vi "_Custom Device Channel.vi"(8 "error in (no error)":errorcluster, 11 "Node Ptr":u64) -> (0 "error out":errorcluster)   [LabVIEW 2020]
uses:
  5565/Source Code/NI VeriStand/Shared/NIVS_Shared.lvlib
  5565/Source Code/NI VeriStand/System Explorer/Communication Layer/Communication.lvlib
  5565/Source Code/NI VeriStand/System Explorer/Communication Layer/FGVActions.ctl
  5565/Source Code/NI VeriStand/Shared/System Storage/Tree Storage/Tree Storage.lvlib
  5565/Source Code/NI VeriStand/System Explorer/System Explorer Framework/System Explorer Framework.lvlib
  5565/Source Code/NI VeriStand/System Explorer/System UI VIs/Custom Device/Custom Device.lvlib
  5565/Source Code/NI VeriStand/Shared/System Storage/Target Sections/Custom Devices/Custom Devices Storage.lvlib
  5565/Source Code/NI VeriStand/Shared/System Storage/Target System Storage/Target System Storage.lvlib
  5565/Source Code/NI VeriStand/Shared/System Storage/Target System Storage/Channel Bitfield Settings.ctl
  5565/Source Code/NI VeriStand/System Explorer/System Explorer Framework/Section Divider.ctl
panel:
  in  "Default Value":dbl
  out "Channel Settings":i32(listbox)
  in  "Channel Settings":T1={"Section Name"="Custom Device Channel Specification"}
  out "Name":string
  in  "Description":string
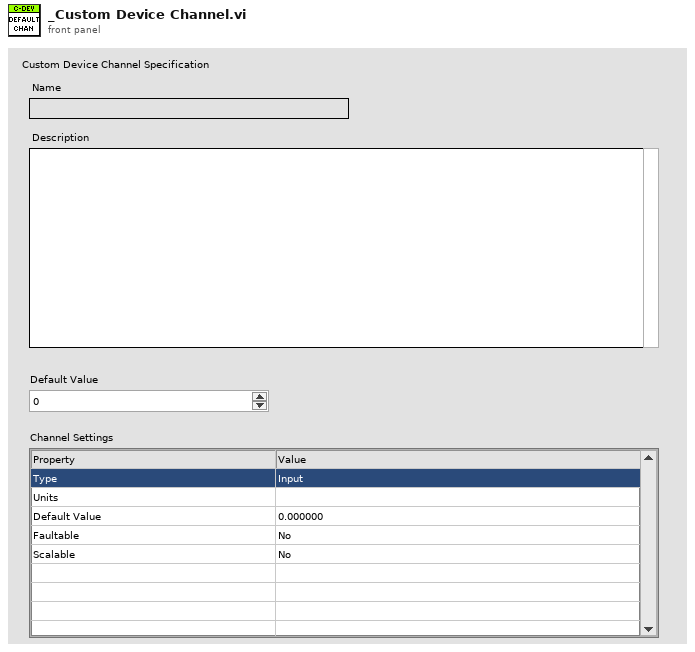
[diagram p1: front panel]
types:
  T1 = typedef "System Explorer Framework.lvlib/Section Divider.ctl" = cluster{"Section Name":string}
  T2 = typedef "Communication.lvlib/FGVActions.ctl" = enum16{"Generate Event", "Get Event Ref", "Create Event", "Destroy"}
  T3 = typedef "NIVS_DataStorage.lvlib/BaseNodeType.ctl" = refnum<k24>
  T4 = typedef "Target System Storage.lvlib/Channel Bitfield Settings.ctl" = enum16{"Read Access", "Write Access", "Faultable", "Scalable"}
  T5 = typedef "Target System Storage.lvlib/Channel Info.ctl" = cluster{"PreScaled Units":string, "Dims":T6, "Def.Value":dbl[], "Bitfield":u32}
  T6 = typedef "Target System Storage.lvlib/Channel Dimensions.ctl" = cluster{"Rows":i32, "Cols":i32}
  T7 = typedef "Communication.lvlib/General Communication Action.ctl" = enum16{"Event structure", "Unsaved", "Release FP Cursor", "Set FP Cursor Busy", "Refresh (Flood)", "Refresh (Add)", "Refresh (Add no highlight)", "Refresh (Repopulate certain node)", "Refresh (Update)", "Refresh (Delete)", "Refresh (Delete no highlight)", "Refresh (Rename)", "Refresh (Move)", "Refresh (Move no highlight)", "Refresh (no highlight)", "Refresh (CD)", "Refresh (single nodes)", "Stop", "GW_WD: Save", "GW_WD: Add Items", "GW_WD: Add Items (no highlight)", "GW_WD: Add Item (CD)", "GW_WD: Update Items", "GW_WD: Delete Item", "GW_WD: Delete Item (no highlight)", "GW_WD: Force Delete Item (no highlight)", "GW_WD: Force Delete Item (no highlight - requested item only)", "GW_WD: Force Delete Item (no highlight - requested item only / Skip Action VI)", "GW_WD: Rename Item", "GW_WD: Move Item", "GW_WD: Repopulate Node", "GW_WD: Load Data from Disk", "GW_WD: Import Data", "GW_WD: New", "GW_WD: Action on Save", "GW_WD: Action on System Shutdown", "GW_WD: Ask save SDF", "GW_WD: Add Revision", "GW_WD: Filter Stop", "GW_WD: Open", "GW_WD: Action on Load", "GW_WD: Save as...", "GW_WD: Deploy", "GW_WD: Close System Explorer", "GW_WD: Current page commit changes", "GW_WD: Current page shutdown", "GW_WD: Add Rev History", "GW_WD: Wait on Action Load", "GW_WD: Signalize Load is Done", "GW_WD: Open File", "GW_WD: Wait on Action Save", "GW_WD: Wait on Action Delete", "GW_WD: Signalize Action Save is Done", "GW_WD: Signalize Action Delete is Done", "GW_WD: Hide Progress Dialog", "GW_WD: Show Progress Dialog", "Delete Cancelled", "GW_WD: Relaunch Page", "GW_WD: Add Item (CD no highlight)", "GW_WD: Activate Progress Window", "GW_WD: Close Progress Window", "GW_WD: Buffering Enabled", "GW_WD: Commit Changes", "GW_WD: Delete Item (notification)", "GW_WD: Force Delete Item (no highlight - notification)", "Page: Send Button ID", "GW_WD: Copy", "GW_WD: Cut", "GW_WD: Paste", "GW_WD: Warning", "GW_WD: Wait on Action Paste", "GW_WD: Signalize Action Paste is Done", "GW_WD: Items Added (highlight)", "GW_WD: Items Added (no highlight)", "GW_WD: Items Added (no highlight / skip action VI)", "GW_WD: Items Added (repopulate certain node)", "GW_WD: Launch Busy Dialog Data Storage", "GW_WD: Stop Busy Dialog Data Storage", "Enable Dynamic Button", "Disable Dynamic Button", "GW_WD: Items Deleted", "GW_WD: Items Deleted (no highlight)", "Insert VI Into SubPanel", "Highlight item", "Update Error Count"}
  T8 = typedef "Communication.lvlib/Listener.ctl" = enum16{"ALL", "System Explorer", "SubPanel VI", "Dialog VI", "Action VI", "GW_WD", "Individual Listener"}
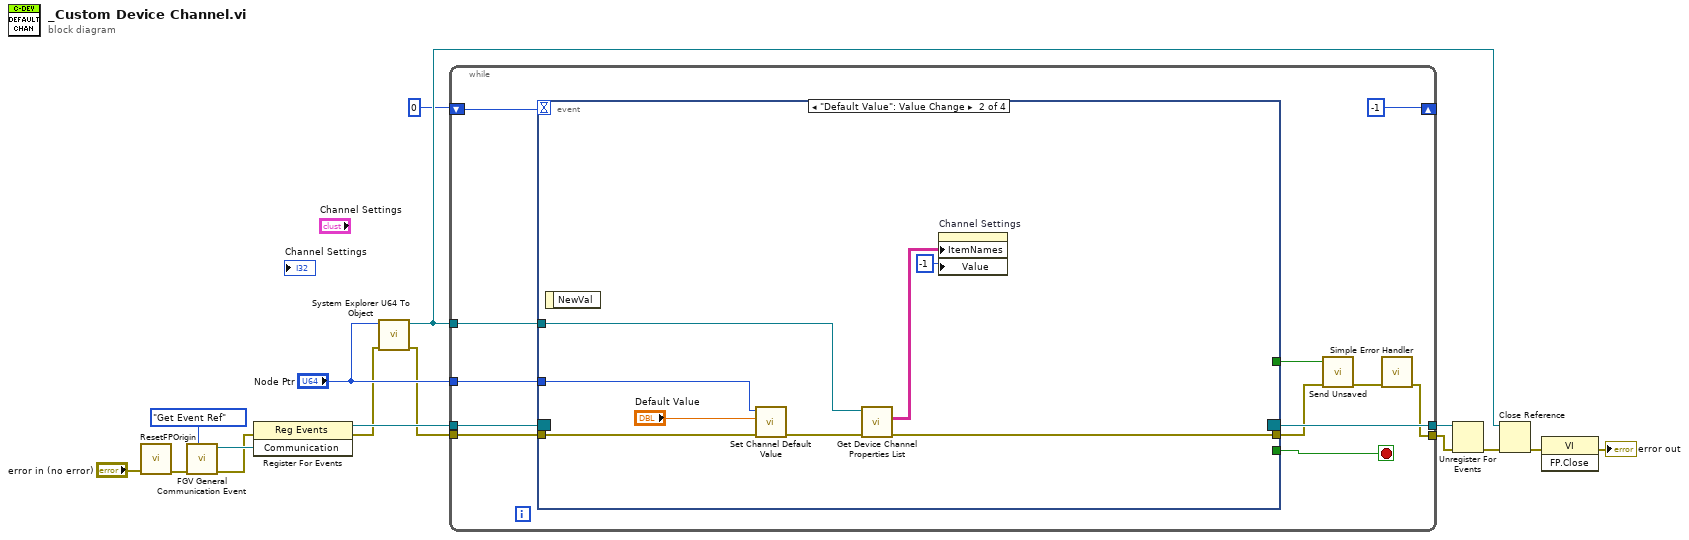
[diagram p0: block diagram]
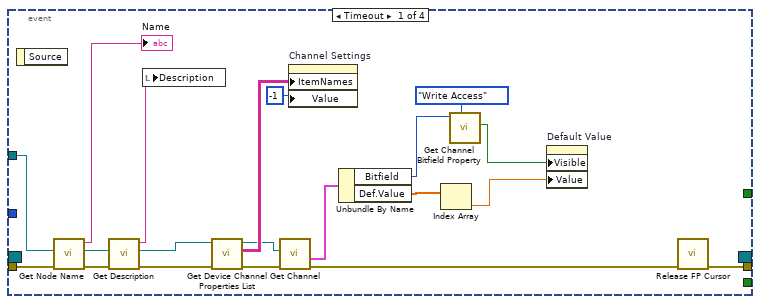
[diagram p2: hidden frame]
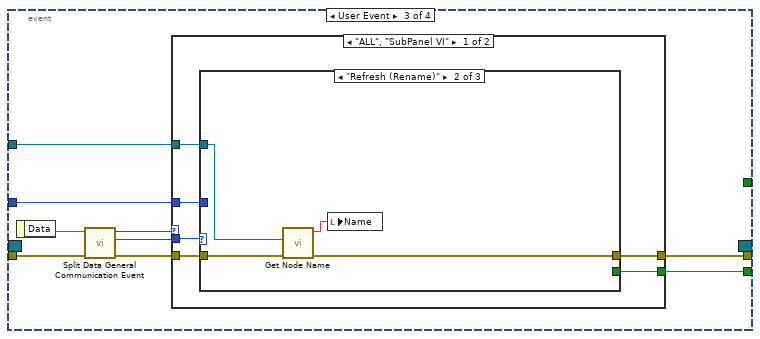
[diagram p3: hidden frame]
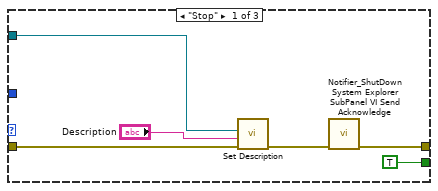
[diagram p4: hidden frame]
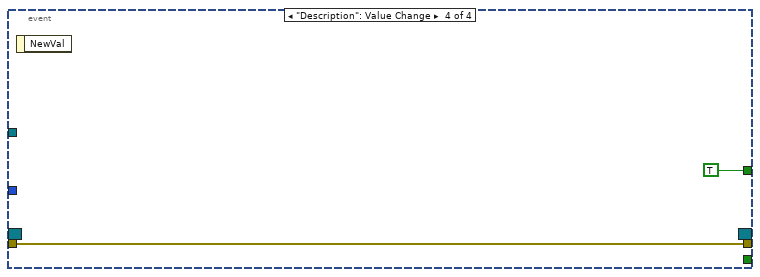
[diagram p7: hidden frame]
diagram:
  n1 = call "ResetFPOrigin.vi"("error in (no error)"="error in (no error)") -> ("error out"=w8:errorcluster)  [unwired: 1 in, 9 out]
  n2 = call "FGV General Communication Event.vi"("Action"=FGVActions."Get Event Ref", "error in (no error)"=w8) -> ("error out"=w11:errorcluster, "Communication"=w12:refnum<user-event>)  [unwired: 1 in, 7 out]
  n3 = register-events(error in=w11, w12) -> (reference out=w10:refnum<event-registration>, error out=w3:errorcluster)  [unwired: 1 in]
  n4 = call "System Explorer U64 To Object.vi"("error in (no error)"=w3, "Node Ptr"="Node Ptr") -> ("error out"=w2:errorcluster, "NodeObject"=w4:T3)  [unwired: 7 in, 1 out]
  n5 = while {
    tunnel: [w28] -> w16
    tunnel: [w27] -> w15
    tunnel: w2 -> [w26]
    tunnel: w10 -> [w25]
    tunnel: "Node Ptr" -> [w23]
    tunnel: w4 -> [w19]
    shift-right: [-1] -> _
    shift-left: 0 -> [w18]
    stop <- w24 stop-if-true
    n6 = event shown="[1] \"Default Value\": Value Change" {
      selector: w25 -> [_ _ _ _]
      dyn-events: [_ _ _ _] -> w28
      timeout: w18 -> [_ _ _ _]
      tunnel: w26 -> [w48 w56 w63 w84]
      tunnel: [_ _ w65 _] -> w24
      tunnel: [w47 w50 w64 w84] -> w21
      tunnel: w23 -> [_ w55 w58 _]
      tunnel: [_ _ _ TRUE] -> w20
      tunnel: w19 -> [w42 w49 w57 _]
      event Timeout {
        n7 = event-data() -> ()  [unwired: 2 out]
        n8 = call "Get Node Name.vi"("error in (no error)"=w48, "BaseNdType"=w42) -> ("error out"=w40:errorcluster, "BaseNdType"=w41:T3, "Node Name"=→"Name":string)  [unwired: 7 out]
        n9 = call "Get Description.vi"("error in (no error)"=w40, "BaseNdType in"=w41) -> ("error out"=w38:errorcluster, "BaseNdType out"=w37:T3, "Description"=w39:string)  [unwired: 6 in, 1 out]
        n10 = local write "Description"(w39) -> ()
        n11 = call "Get Device Channel Properties List.vi"("error in (no error)"=w38, "Channel Ref in"=w37) -> ("error out"=w35:errorcluster, "Properties List"=w44:string[][], "Channel Ref out"=w36:T3)  [unwired: 7 out]
        n12 = call "Get Channel.vi"("error in (no error)"=w35, "Channel"=w36) -> ("error out"=w34:errorcluster, "Channel Info"=w33:T5)  [unwired: 6 in, 2 out]
        n13 = property on="Channel Settings" class="MCListbox (strict)"("ItemNames"=w44, "Value"=-1 ("Channel Settings")) -> ()  [unwired: 2 in, 2 out]
        n14 = Unbundle By Name(w33) -> ("Bitfield"=w30:u32, "Def.Value"=w43:dbl[])
        n15 = Index Array(array=w43) -> (element=w32:dbl)  [unwired: 1 in]
        n16 = call "Get Channel Bitfield Property.vi"("Bitfield Setting"=Channel_Bitfield_Settings."Write Access", "Channel Bitfield"=w30) -> ("Value"=w29:bool)  [unwired: 9 out]
        n17 = property on="Default Value" class="DigNum (strict)"("Visible"=w29, "Value"=w32) -> ()  [unwired: 2 in, 2 out]
        n18 = call "Release FP Cursor.vi"("error in (no error)"=w34) -> ("error out"=w47:errorcluster)  [unwired: 10 out]
      }
      event "Default Value": Value Change {
        n19 = event-data() -> ()  [unwired: 2 out]
        n20 = call "Set Channel Default Value.vi"("error in (no error)"=w56, "Default Value"="Default Value", "Channel Ref in"=w55) -> ("error out"=w51:errorcluster)  [unwired: 8 out]
        n21 = call "Get Device Channel Properties List.vi"("error in (no error)"=w51, "Channel Ref in"=w49) -> ("error out"=w50:errorcluster, "Properties List"=w52:string[][])  [unwired: 8 out]
        n22 = property on="Channel Settings" class="MCListbox (strict)"("ItemNames"=w52, "Value"=-1 ("Channel Settings")) -> ()  [unwired: 2 in, 2 out]
      }
      event User Event {
        n23 = event-data() -> ("Data"=w62:string)  [unwired: 1 out]
        n24 = call "Split Data General Communication Event.vi"("error in"=w63, "Data"=w62) -> ("error out"=w61:errorcluster, "Action"=w59:T7, "Listener"=w60:T8)  [unwired: 7 out]
        n25 = case shown="\"ALL\", \"SubPanel VI\"" w60 {
          tunnel: w61 -> [w70 w83]
          tunnel: w59 -> [w71 _]
          tunnel: [w69 _] -> w65
          tunnel: [w68 w83] -> w64
          tunnel: w58 -> [w67 _]
          tunnel: w57 -> [w66 _]
          frame "ALL", "SubPanel VI" {
            n26 = case shown="\"Refresh (Rename)\"" w71 {
              tunnel: w70 -> [w73 w81 w82]
              tunnel: [w77 w79 w82] -> w68
              tunnel: [TRUE _ _] -> w69
              tunnel: w67 -> [_ _ _]
              tunnel: w66 -> [w75 w78 _]
              frame "Stop" {
                n27 = call "Set Description.vi"("error in (no error)"=w73, "Description"="Description", "BaseNdType in"=w75) -> ("error out"=w72:errorcluster)  [unwired: 6 in, 2 out]
                n28 = call "Notifier_ShutDown System Explorer SubPanel VI Send Acknowledge.vi"("error in (no error)"=w72) -> ("error out"=w77:errorcluster)  [unwired: 1 in, 9 out]
              }
              frame "Refresh (Rename)" {
                n29 = call "Get Node Name.vi"("error in (no error)"=w81, "BaseNdType"=w78) -> ("error out"=w79:errorcluster, "Node Name"=w80:string)  [unwired: 8 out]
                n30 = local write "Name"(w80) -> ()
              }
              frame Default {
              }
            }
          }
          frame Default {
          }
        }
      }
      event "Description": Value Change {
        n31 = event-data() -> ()  [unwired: 2 out]
      }
    }
    n32 = call "Send Unsaved.vi"("error in (no error)"=w21, "Send unsaved? (T)"=w20) -> ("error out"=w22:errorcluster)  [unwired: 9 out]
    n33 = call <vilib>:"Simple Error Handler.vi"("error in (no error)"=w22) -> ("error out"=w27:errorcluster)  [unwired: 1 in, 7 out]
  }
  n34 = Unregister For Events(event registration refnum=w16, error in=w15) -> (error out=w6:errorcluster)
  n35 = Close Reference(reference=w4, error in (no error)=w6) -> (error out=w5:errorcluster)
  n36 = invoke class="VI" method="FP.Close"(error in=w5) -> (error out=→"error out":errorcluster)  [unwired: 2 in, 2 out]
